vi "ThreePhasePLL_src.vi"(5 "PLLrange":T2={"output high (Inf)"=inf, "output low (-Inf)"=-inf}, 6 "reset":bool, 7 "PLLgains":T3 {"proportional gain" step=0.125}, 8 "StateIn":T4 {"Phase" format="%#_13g"}, 9 "GridExpectedFreq":sgl, 10 "dT":sgl, 11 "Vq":sgl) -> (0 "StateOut":T4 {"Phase" format="%#_13g"}, 1 "PLLactions":T1, 3 "gridFrequency":sgl)   [LabVIEW 2015]
uses:
  AFE/ThreePhasePLLState.ctl
  <vilib>/rvi/Analysis/control/PID/Typedef/niFpgaPID_PIGains.ctl
  <vilib>/rvi/Analysis/control/PID/Typedef/niFpgaPID_OutputRange.ctl
  <vilib>/rvi/Analysis/control/PID/Typedef/niFpgaPID_PIActions.ctl
  <vilib>/rvi/Analysis/control/PID/Typedef/niFpgaPID_PIErrors.ctl
  <vilib>/rvi/Analysis/control/PID/Typedef/niFpgaPID_PIState.ctl
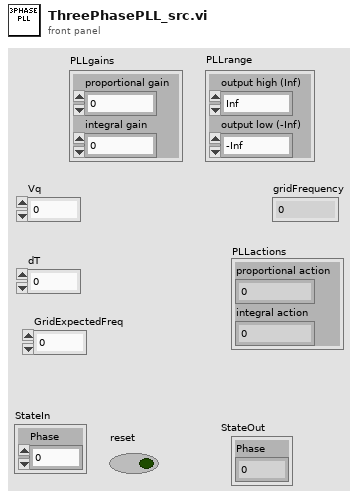
[diagram p1: front panel]
types:
  T1 = typedef "niFpgaPID_PIActions.ctl" = cluster{"proportional action":sgl, "integral action":sgl}
  T2 = typedef "niFpgaPID_OutputRange.ctl" = cluster{"output high (Inf)":sgl, "output low (-Inf)":sgl}
  T3 = typedef "niFpgaPID_PIGains.ctl" = cluster{"proportional gain":sgl, "integral gain":sgl}
  T4 = typedef "ThreePhasePLLState.ctl" = cluster{"Phase":sgl}
  T5 = typedef "niFpgaPID_PIState.ctl" = cluster{"uI(k-1)":sgl, "e(k-1)":sgl, "output (k-1)":sgl}
  T6 = typedef "niFpgaPID_PIErrors.ctl" = cluster{"error":sgl, "error with beta":sgl}
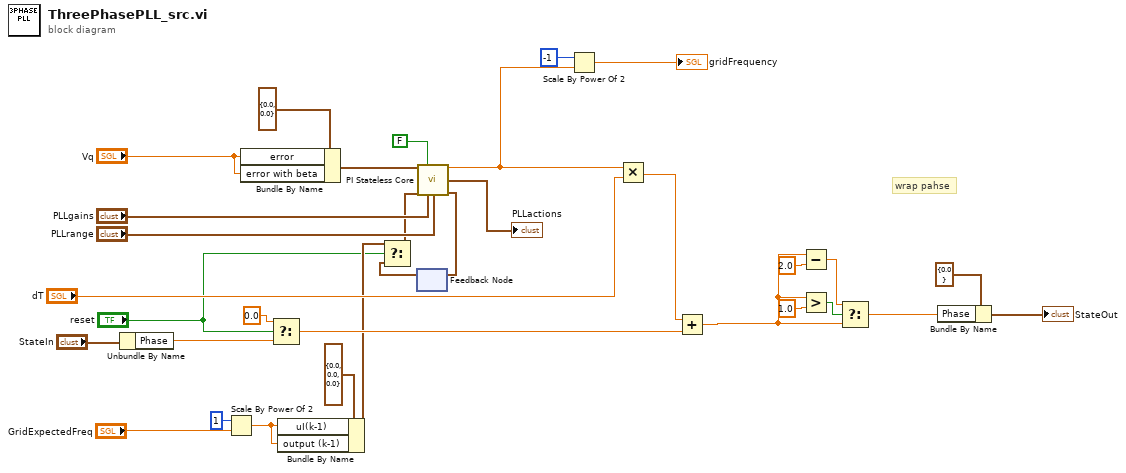
[diagram p0: block diagram]
diagram:
  # "wrap pahse"
  n1 = Unbundle By Name("StateIn") -> ("Phase"=w18:sgl)
  n2 = Scale By Power Of 2(n=i16 1, x="GridExpectedFreq") -> (x*2^n=w4:sgl)
  n3 = Bundle By Name(cluster=T6 {"error"=0.0, "error with beta"=0.0} ("errors"), "error"="Vq", "error with beta"="Vq") -> (w30:T6)
  n4 = Select(t=sgl 0.0, s="reset", f=w18) -> (s? t:f=w17:sgl)
  n5 = Bundle By Name(cluster=T5 {"uI(k-1)"=0.0, "e(k-1)"=0.0, "output (k-1)"=0.0} ("state out"), "uI(k-1)"=w4, "output (k-1)"=w4) -> (w8:T5)
  n6 = feedback #1() -> (w7:T5)  [unwired: 1 in]
  n7 = Select(t=w8, s="reset", f=w7) -> (s? t:f=w6:T5)
  n8 = call "PI Stateless Core"("errors"=w30, "reset? (F)"=FALSE, "state in"=w6, "gains"="PLLgains", "output range"="PLLrange") -> ("output"=w13:sgl, "actions"=→"PLLactions":T1, "state out"=w29:T5)  [unwired: 7 in, 1 out]
  n9 = feedback-in #1(w29) -> ()
  n10 = Scale By Power Of 2(n=i16 -1, x=w13) -> (x*2^n=→"gridFrequency":sgl)
  n11 = Multiply(x=w13, y="dT") -> (x*y=w15:sgl)
  n12 = Add(x=w15, y=w17) -> (x+y=w2:sgl)
  n13 = Subtract(x=w2, y=sgl 2.0) -> (x-y=w22:sgl)
  n14 = Greater?(x=w2, y=sgl 1.0) -> (0:w21:bool)
  n15 = Select(t=w22, s=w21, f=w2) -> (s? t:f=w1:sgl)
  n16 = Bundle By Name(cluster=T4 {"Phase"=0.0} ("StateOut"), "Phase"=w1) -> (→"StateOut":T4)
